vi "Dashboard_event.vi"(8 "error in":errorcluster, 9 "array_enc_in":T1, 10 "Estado":T6, 11 "New_data?":bool) -> (0 "error out":errorcluster, 2 "Dashboard_userEvent_out":refnum<user-event>)   [LabVIEW 2026]
uses:
  Control/Ctrl_GuiEvent.ctl
  Control/Ctrl_Array_Enc_Out.ctl
  Control/Ctr_Enc_Values.ctl
  Control/Ctrl_datos6motores_final.ctl
  Control/Ctrl_Motores_Valores.ctl
  Control/Ctrl_Errores.ctl
  Control/Cluster_Dashboard.ctl
  Control/Ctrl_Dashboard_StateMach.ctl
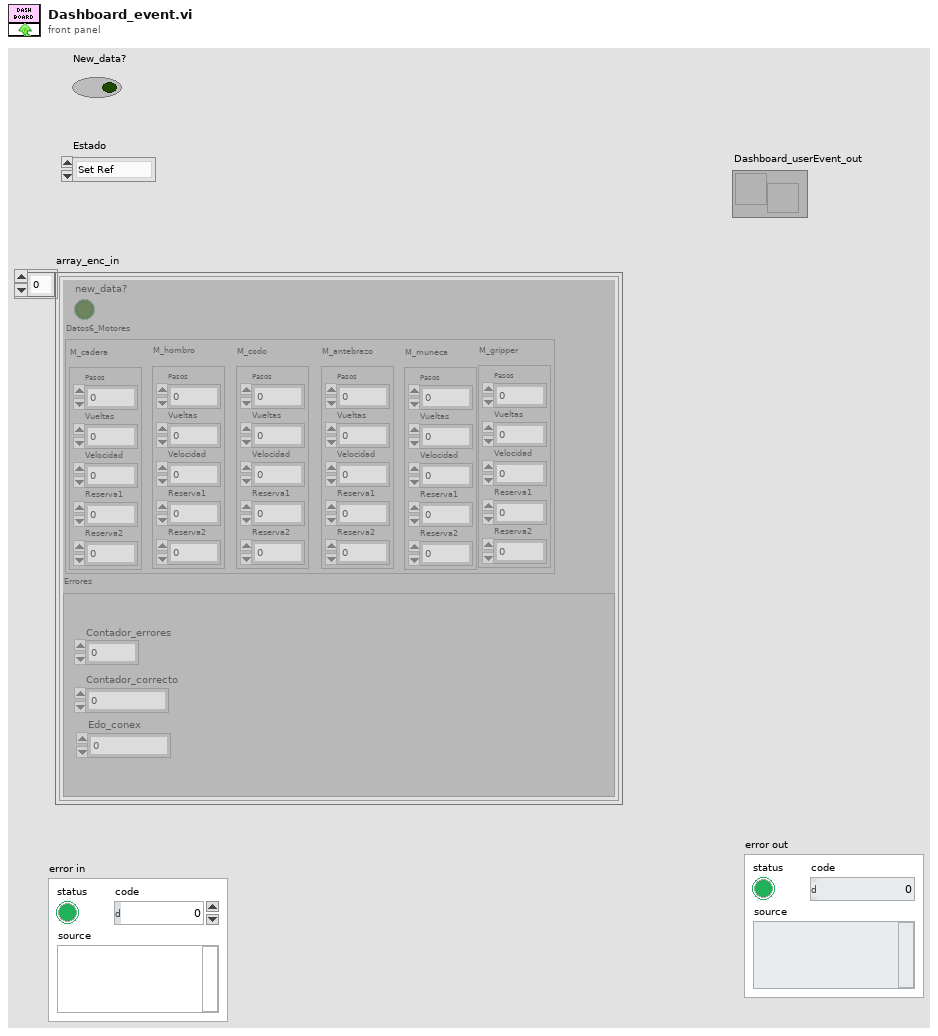
[diagram p1: front panel]
types:
  T1 = typedef "Ctrl_Array_Enc_Out.ctl" = T2[]
  T2 = typedef "Ctr_Enc_Values.ctl" = cluster{"Datos6_Motores":T3, "Errores":T5, "new_data?":bool}
  T3 = typedef "Ctrl_datos6motores_final.ctl" = cluster{"M_cadera":T4, "M_hombro":T4, "M_codo":T4, "M_antebrazo":T4, "M_muneca":T4, "M_gripper":T4}
  T4 = typedef "Ctrl_Motores_Valores.ctl" = cluster{"Pasos":i32, "Vueltas":i16, "Velocidad":dbl, "Reserva1":u8, "Reserva2":u8}
  T5 = typedef "Ctrl_Errores.ctl" = cluster{"Contador_correcto":u32, "Contador_errores":u32, "Edo_conex":u32}
  T6 = typedef "Ctrl_GuiEvent.ctl" = enum16{"Set Ref", "Update Enc", "Stop", "Get Ref"}
  T7 = typedef "Cluster_Dashboard.ctl" = cluster{"Array_encoders":T1, "Estado":T8}
  T8 = typedef "Ctrl_Dashboard_StateMach.ctl" = enum16{"Stop", "Update", "Start"}
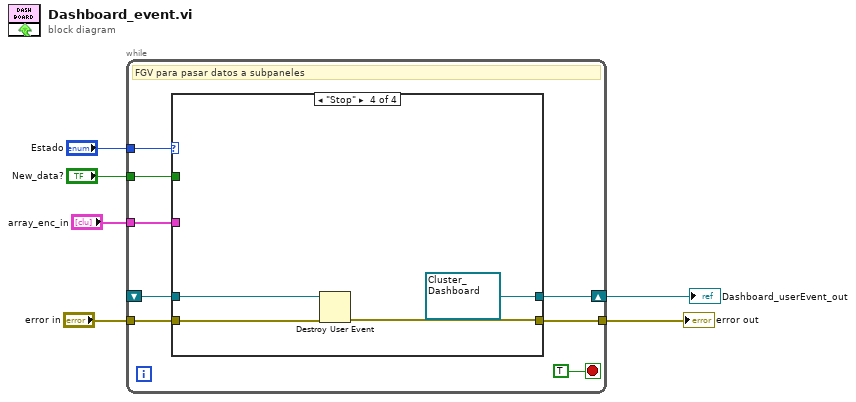
[diagram p0: block diagram]
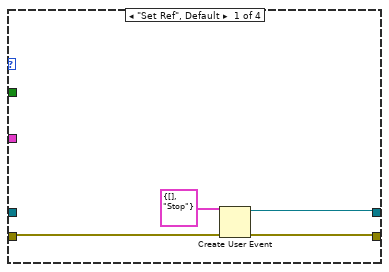
[diagram p2: hidden frame]
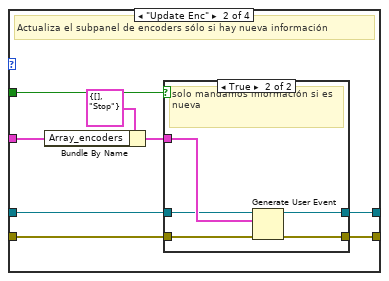
[diagram p3: hidden frame]
diagram:
  n1 = while {
    tunnel: "Estado" -> [w13]
    tunnel: "error in" -> [w12]
    tunnel: [w11] -> w4
    tunnel: "New_data?" -> [w10]
    tunnel: "array_enc_in" -> [w9]
    shift-right: [w7] -> w1
    shift-left: _ -> [w8]
    stop <- TRUE stop-if-true
    # "FGV para pasar datos a subpaneles"
    n2 = case shown="\"Stop\"" w13 {
      tunnel: w12 -> [w15 w26 w35 w39]
      tunnel: [w16 w25 w35 w38] -> w11
      tunnel: w10 -> [_ w24 _ _]
      tunnel: w9 -> [_ w22 _ _]
      tunnel: w8 -> [_ w20 w34 w36]
      tunnel: [w17 w19 w34 refnum<user-event> refnum ("Dashboard_userEvent_in")] -> w7
      frame "Set Ref", Default {
        n3 = Create User Event(user event datatype=T7 {"Array_encoders"=[], "Estado"=enum."Stop"} ("Cluster_Dashboard"), error in=w15) -> (user event=w17:refnum<user-event>, error out=w16:errorcluster)
      }
      frame "Update Enc" {
        # "Actualiza el subpanel de encoders sólo si hay nueva información"
        n4 = Bundle By Name(cluster=T7 {"Array_encoders"=[], "Estado"=enum."Stop"}, "Array_encoders"=w22) -> (w21:T7)
        n5 = case shown="True" w24 {
          tunnel: w26 -> [w28 w33]
          tunnel: [w28 w32] -> w25
          tunnel: w21 -> [_ w31]
          tunnel: w20 -> [w27 w30]
          tunnel: [w27 w29] -> w19
          frame False {
            # "no hay información nueva"
          }
          frame True {
            # "solo mandamos información si es nueva"
            n6 = Generate User Event(user event=w30, event data cluster=w31, error in=w33) -> (user event out=w29:refnum<user-event>, error out=w32:errorcluster)  [unwired: 1 in]
          }
        }
      }
      frame "Get Ref" {
      }
      frame "Stop" {
        n7 = Destroy User Event(user event=w36, error in=w39) -> (error out=w38:errorcluster)
      }
    }
  }
  "error out" <- w4
  "Dashboard_userEvent_out" <- w1
